vi "treeScan.vi"() -> ()   [LabVIEW 2017]
uses:
  <vilib>/MDSplus/Library/MDSplus.lvlib
panel:
  out "数值":i32
  out "数组":string[](array[string])
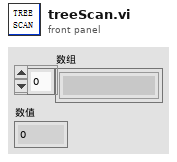
[diagram p1: front panel]
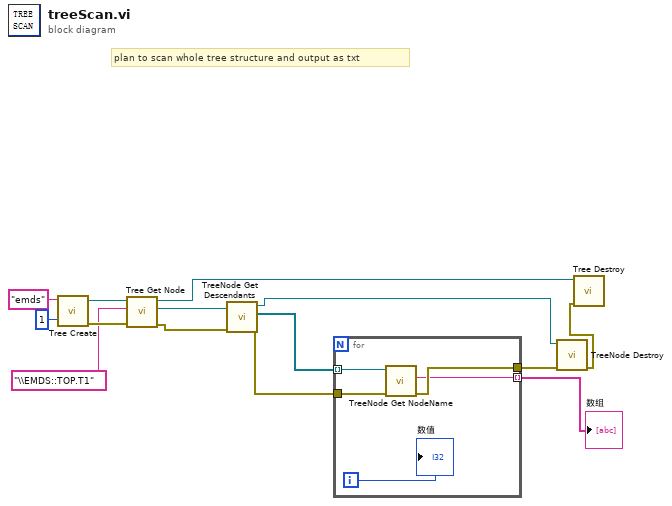
[diagram p0: block diagram]
diagram:
  # "plan to scan whole tree structure and output as txt"
  n1 = call <vilib>:"Tree Create.vi"("Shot"=1, "Name"="emds") -> ("error out"=w11:errorcluster, "Tree DVR out"=w14:refnum<data-value>)  [unwired: 8 in]
  n2 = call <vilib>:"Tree Get Node.vi"("error in (no error)"=w11, "Path"="\\EMDS::TOP.T1", "Tree DVR in"=w14) -> ("error out"=w9:errorcluster, "Node out"=w3:refnum<data-value>, "Tree DVR out"=w4:refnum<data-value>)  [unwired: 6 in]
  n3 = call <vilib>:"TreeNode Get Descendants.vi"("error in (no error)"=w9, "TreeNode DVR in"=w3) -> ("error out"=w7:errorcluster, "TreeNodeArray"=w8:refnum<data-value>[], "TreeNode DVR out"=w6:refnum<data-value>)  [unwired: 7 in]
  n4 = for {
    tunnel: w8 -> [w18] mode=indexing
    tunnel: w7 -> [w17]
    tunnel: [w16] -> w2
    tunnel: [w15] -> w1 mode=indexing
    i -> [w19]
    n5 = call <vilib>:"TreeNode Get NodeName.vi"("error in (no error)"=w17, "TreeNode DVR in"=w18) -> ("error out"=w16:errorcluster, "NodeName"=w15:string)  [unwired: 7 in, 1 out]
    "数值" <- w19
  }
  "数组" <- w1
  n6 = call <vilib>:"TreeNode Destroy.vi"("error in (no error)"=w2, "TreeNode DVR in"=w6) -> ("error out"=w5:errorcluster)  [unwired: 9 in]
  n7 = call <vilib>:"Tree Destroy.vi"("error in (no error)"=w5, "Tree DVR in"=w4) -> ()  [unwired: 9 in, 1 out]
